vi "driveOffTest.vi"(10 "Trigger":bool) -> (2 "Drive Power":dbl)   [LabVIEW 2018]
panel:
  in  "Width (sec)":dbl=1.0
  in  "Go":dbl=0.8
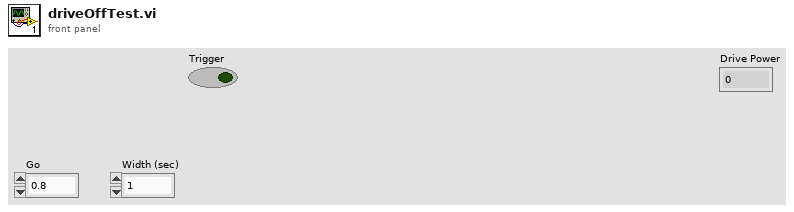
[diagram p1: front panel]
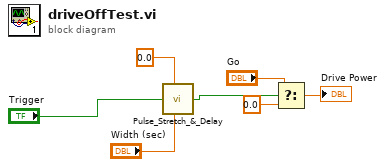
[diagram p0: block diagram]
diagram:
  n1 = call <userlib>:"Pulse_Stretch_&_Delay.vi"("Delay (sec)"=0.0, "In"="Trigger", "Width (sec)"="Width (sec)") -> ("Out"=w7:bool)  [unwired: 2 in]
  n2 = Select(t="Go", s=w7, f=0.0) -> (s? t:f=→"Drive Power":dbl)
